vi "logstring_lua.vi"(5 "LuaVIEW reference":T1) -> (15 "error out":errorcluster)   [LabVIEW 2012]
doc: "This function is NOT for general use. It logs a string to a tag of the current database, but normally the <code>StringTag.write</code> function/method must be used for that. This function should be used only for those few logging requirements that must keep on working when datalogging is not active. This is desirable for logging errors or warnings to a string tag: before the system has reached the \"datalogging\" runlevel it must succeed in lots of configuration and initialisation actions that are prone to throwing errors that, when they do occur, should be logged somewhere. To support this requirement, this function is implemented such that it can log a string irrespective of whether the database is live or not.\n\nWhen the current database is live, the normal buffered logging mechanism is used. Otherwise the string tag log is directly appended to without in-memory buffering. This function is smart enough to keep on functioning when the system has only partially initialised towards or cleaned up from a live logging state: when the database is live, it first tries buffered string writing and, when that fails, it attempts the direct approach.\nParameters:\nstr:tag, name of the tag.\nstr:string, string to log.\n[num:time], timestamp for logged string, if omitted the current time is used.\nErrors:\nDatabases module not initialised.\nCurrent database is locked.\nTag does not exist.\nTag is not a string tag."
uses:
  luaview/typedefs/t_LuaVIEW Reference.ctl
  luaview/subvis/private/LuaVIEW Pull (string).vi
  luaview/subvis/private/LuaVIEW Pull (number).vi
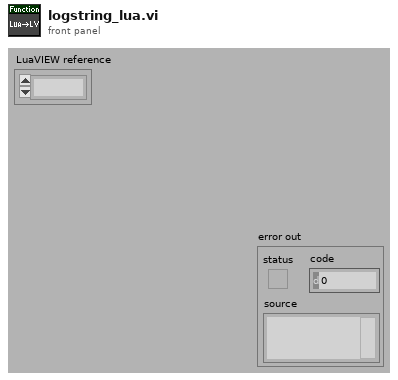
[diagram p1: front panel]
types:
  T1 = typedef "t_LuaVIEW Reference.ctl" = refnum<k1>
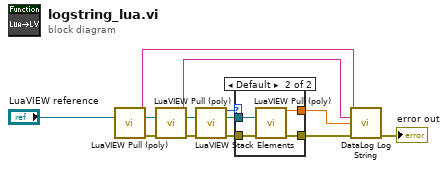
[diagram p0: block diagram]
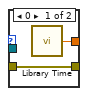
[diagram p2: hidden frame]
diagram:
  n1 = call-poly "LuaVIEW Pull (poly).vi"("LuaVIEW reference in"="LuaVIEW reference") -> ("string"=w3:string, "LuaVIEW reference out"=w6:T1, "error out"=w7:errorcluster)  [unwired: 12 in]
  n2 = call-poly "LuaVIEW Pull (poly).vi"("LuaVIEW reference in"=w6, "error in (no error)"=w7) -> ("string"=w2:string, "LuaVIEW reference out"=w9:T1, "error out"=w8:errorcluster)  [unwired: 11 in]
  n3 = call "LuaVIEW Stack Elements.vi"("LuaVIEW reference in"=w9, "error in (no error)"=w8) -> ("elements"=w10:i32, "LuaVIEW reference out"=w11:T1, "error out"=w12:errorcluster)  [unwired: 11 in]
  n4 = case shown="Default" w10 {
    tunnel: [w15 w19] -> w5
    tunnel: [w14 w18] -> w1
    tunnel: w11 -> [_ w17]
    tunnel: w12 -> [w15 w16]
    frame 0 {
      n5 = call "Library Time.vi"() -> ("time"=w14:dbl)  [unwired: 1 in]
    }
    frame Default {
      n6 = call-poly "LuaVIEW Pull (poly).vi"("LuaVIEW reference in"=w17, "error in (no error)"=w16) -> ("number"=w18:dbl, "error out"=w19:errorcluster)  [unwired: 11 in, 1 out]
    }
  }
  n7 = call "DataLog Log String.vi"("tag"=w3, "string"=w2, "time"=w1, "error in (no error)"=w5) -> ("error out"=→"error out":errorcluster)  [unwired: 11 in]
